vi "Action Reset Min-Max.vi"(0 "VISA resource name":refnum<visa-resource-name>, 7 "Reset Min/Max (T: Reset)":bool=TRUE, 11 "error in (no error)":errorcluster) -> (4 "VISA resource name out":refnum<visa-resource-name>, 15 "error out":errorcluster)   [LabVIEW 2012, in "Lake Shore Cryotronics 218.lvlib"]
doc: "This VI resets the minimum and maximum data for all inputs."
uses:
  <instrlib>/Lake Shore Cryotronics 218/Lake Shore Cryotronics 218.lvlib
panel:
  # "Reset\nDon't Reset"
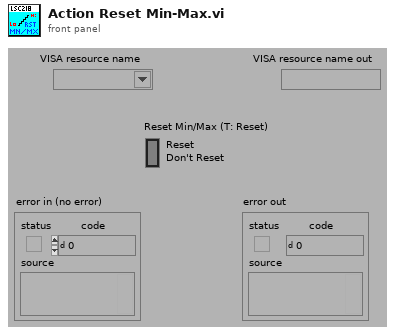
[diagram p1: front panel]
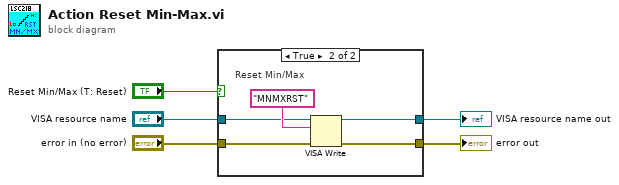
[diagram p0: block diagram]
diagram:
  n1 = case shown="True" "Reset Min/Max (T: Reset)" {
    tunnel: "VISA resource name" -> [w7 w11]
    tunnel: "error in (no error)" -> [w6 w10]
    tunnel: [w7 w9] -> w4
    tunnel: [w6 w8] -> w3
    frame False {
      # "Do not reset Min/Max."
    }
    frame True {
      # "Reset Min/Max"
      n2 = VISA Write(VISA resource name=w11, write buffer="MNMXRST", error in (no error)=w10) -> (VISA resource name out=w9:refnum<visa-resource-name>, error out=w8:errorcluster)  [unwired: 1 out]
    }
  }
  "error out" <- w3
  "VISA resource name out" <- w4
